vi "ModbusSlaveHmi.vi"() -> ()   [LabVIEW 2018, in "ModbusTestSlaveLibrary.lvlib"]
uses:
  ModbusTestSlaveLibrary.lvlib
panel:
  out "Cycle":i32
  in  "Stop":bool
  out "Holding Registry #2 (40002)":u16(slide) scale=0.0..255.0
  in  "Input Registry #2 (30002)":u16(slide) scale=0.0..1023.0
  in  "Input Registry #1 (30001)":u16(slide) scale=0.0..1023.0
  in  "Discrete Input #2 (10002)":bool
  in  "Discrete Input #1 (10001)":bool
  out "Holding Registry #1 (40001)":u16(slide) scale=0.0..255.0
  out "Coil #2 (00002)":bool
  out "Coil #1 (00001)":bool
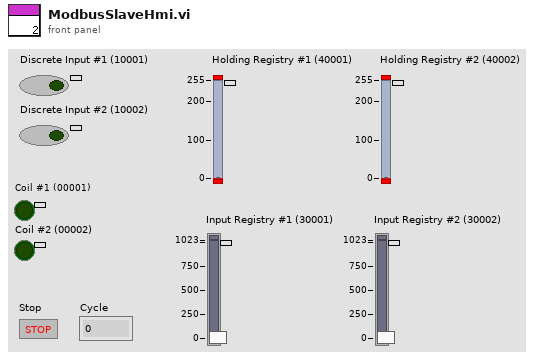
[diagram p1: front panel]
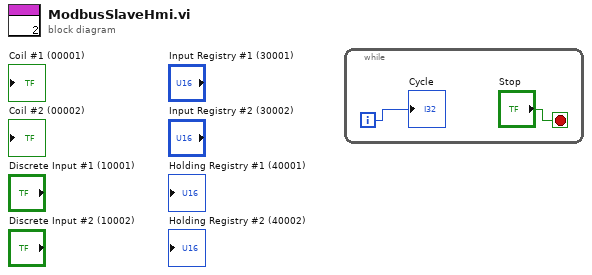
[diagram p0: block diagram]
diagram:
  n1 = while {
    i -> [w2]
    stop <- "Stop" stop-if-true
    "Cycle" <- w2
  }
